vi "Worker Main.vi"() -> ()   [LabVIEW 2013, in "VIChallenge.lvlib"]
uses:
  <vilib>/LabVIEW Hacker/VIChallenge/VIChallenge.lvlib
  <vilib>/LabVIEW Hacker/VIChallenge/Public/Worker State.ctl
  <vilib>/LabVIEW Hacker/LVH-Toolbox/Common/LVH-Common.lvlib
  <vilib>/National Instruments/LabVIEW Interface for Amazon S3/LV Interface for Amazon S3.lvlib
panel:
  out "Iterations":i32
  in  "Stop Button":bool
  out "Error Out":errorcluster
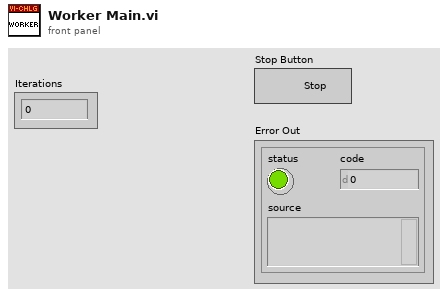
[diagram p1: front panel]
types:
  T1 = typedef "VIChallenge.lvlib/Worker State.ctl" = enum16{"Poll For Job", "Get Source", "Grade", "Notify User"}
  T2 = typedef "VIChallenge.lvlib/VIChallenge Config.ctl" = cluster{"AWS Credentials":T3, "AWS Account Number":string, "SQS Jobs":refnum<class "AWS_SQS.lvclass">, "SQS Status":refnum<class "AWS_SQS.lvclass">, "Source Dir":path, "Working Dir":path, "Output Dir":path, "Archive Dir":path, "job":T4, "Database Ref":T5, "Challenge Dir":path, "Challenges":T6[]}
  T3 = typedef "AWS_Core.lvlib/AWS_AWS Credentials.ctl" = cluster{"AWSAccessKeyId":string, "Secret Key":string}
  T4 = typedef "VIChallenge.lvlib/JSON_job.ctl" = cluster{"job_id":string, "challenge_id":string, "user_id":string, "s3_source_bucket":string, "s3_source_directory":string, "s3_source_filename":string, "status_queue_name":string, "username":string}
  T5 = typedef "NI_Database_API.lvlib/Conn ObjectReference.ctl" = refnum<k1>
  T6 = typedef "VIChallenge.lvlib/Challenge.ctl" = cluster{"General":cluster{"Challenge Id":i32, "Template Path":path, "Solution Path":path, "Primary Score":string, "Score Sort":string}, "Unit Test Framework":cluster{"Enabled Unit Test Templates":path[]}, "VI Analyzer":cluster{"Enabled VI Analyzer Tests":path[]}, "Custom Tests":cluster{"Enabled Custom Tests":path[]}}
  T7 = enum16{"open", "replace", "create", "open or create", "replace or create", "replace or create with confirmation"}
  T8 = typedef "VIChallenge.lvlib/Grader Result.ctl" = cluster{"Id":string, "Score":T9}
  T9 = typedef "VIChallenge.lvlib/Score.ctl" = cluster{"Status":T10, "cpu_time":i32, "max_memory":i32, "style_score":i32, "score0":string, "score1":string, "score2":string, "score3":string, "score4":string, "score5":string}
  T10 = typedef "VIChallenge.lvlib/UTF Status.ctl" = enum16{"Null", "Passed", "Failed", "Error", "Skipped", "Not Processed"}
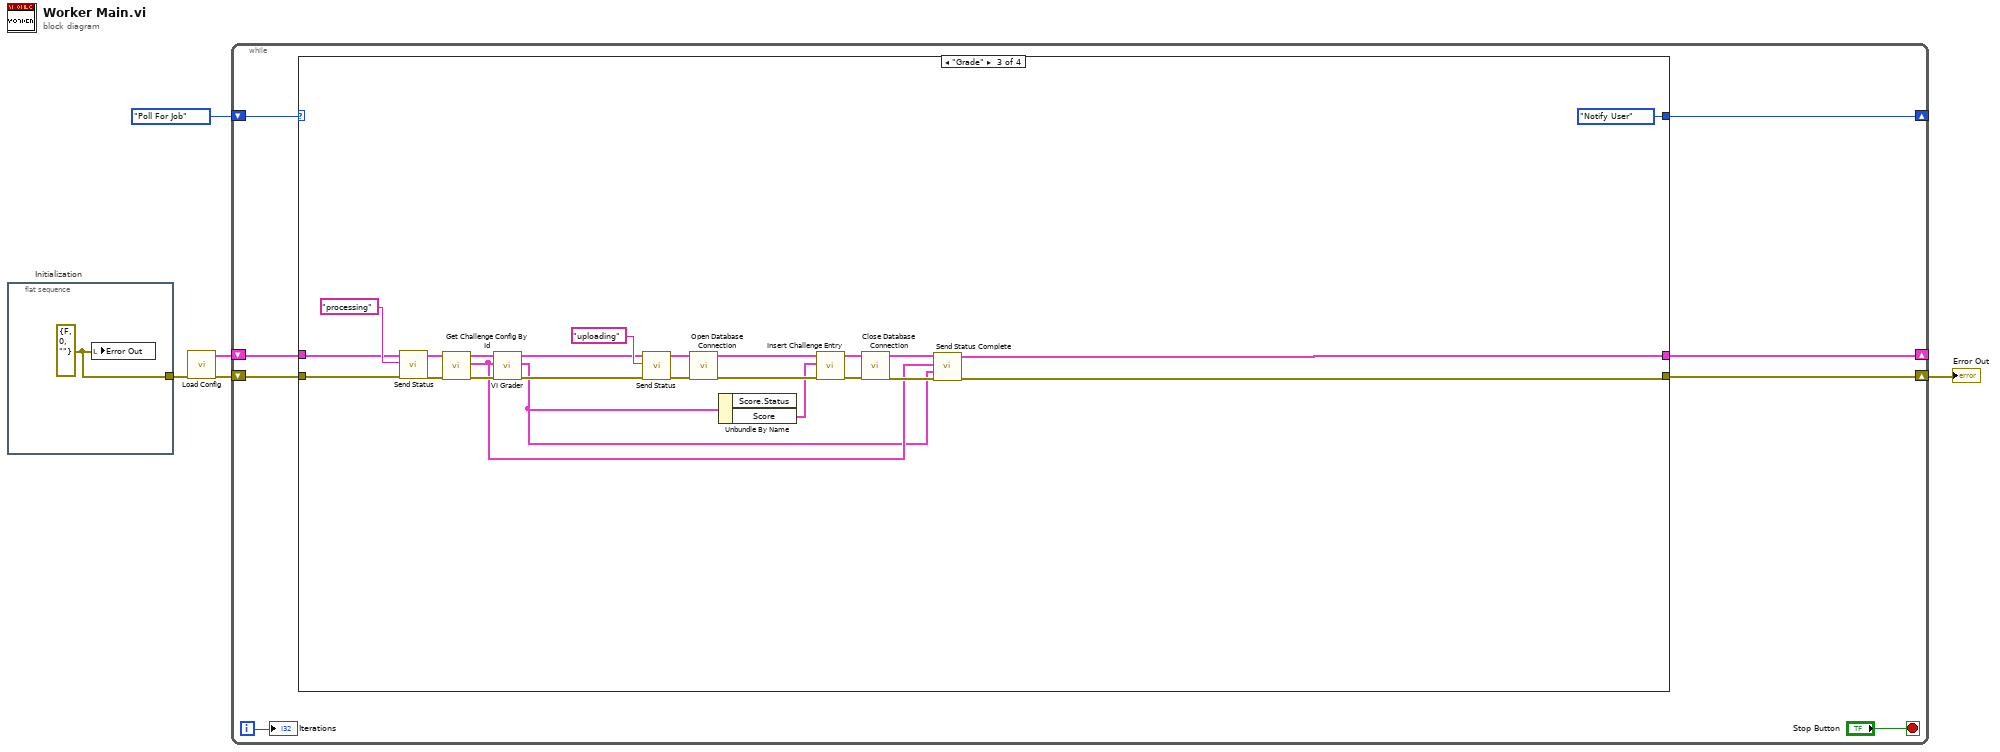
[diagram p0: block diagram]
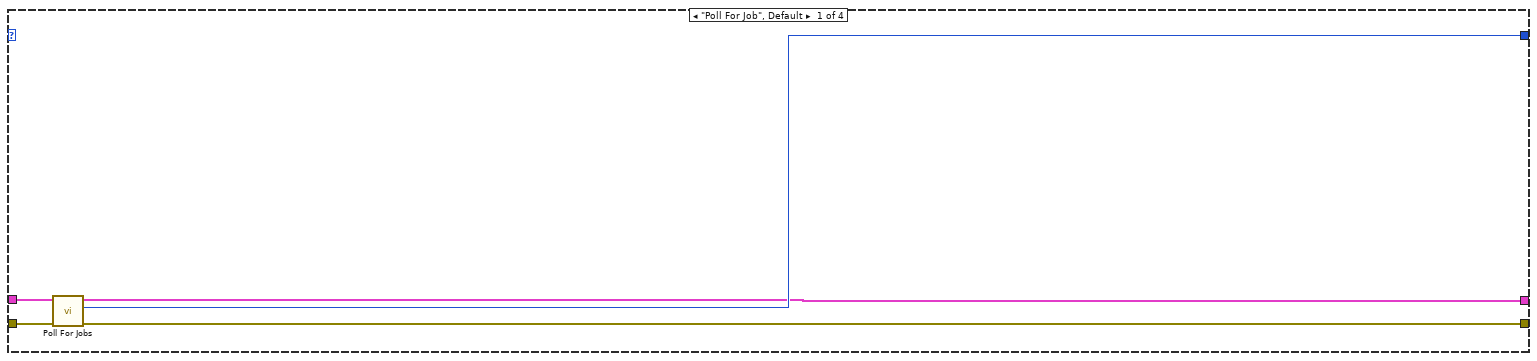
[diagram p2: hidden frame]
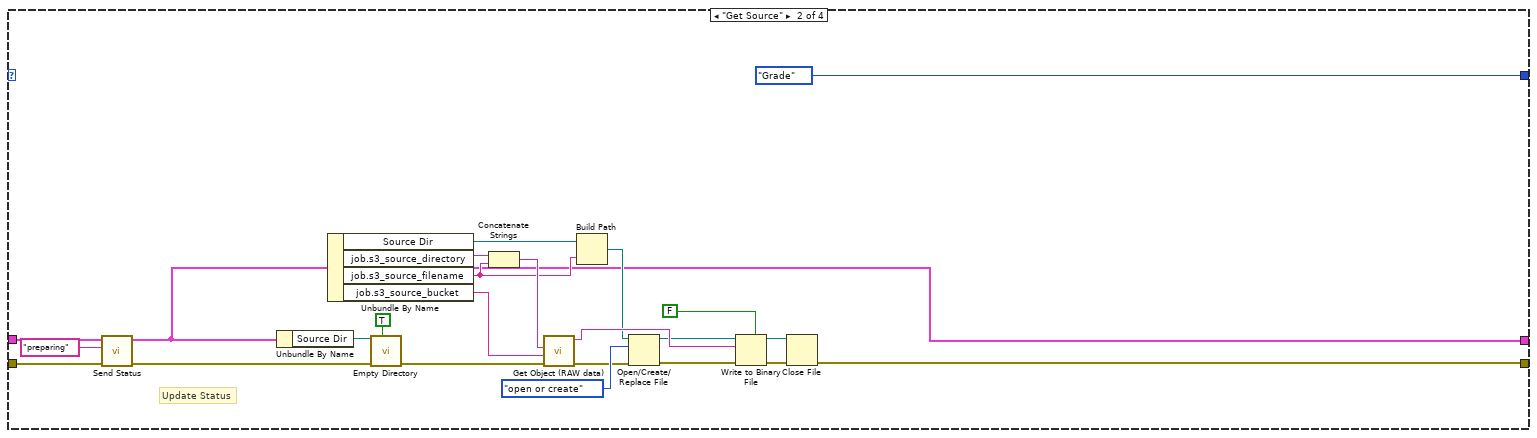
[diagram p3: hidden frame]
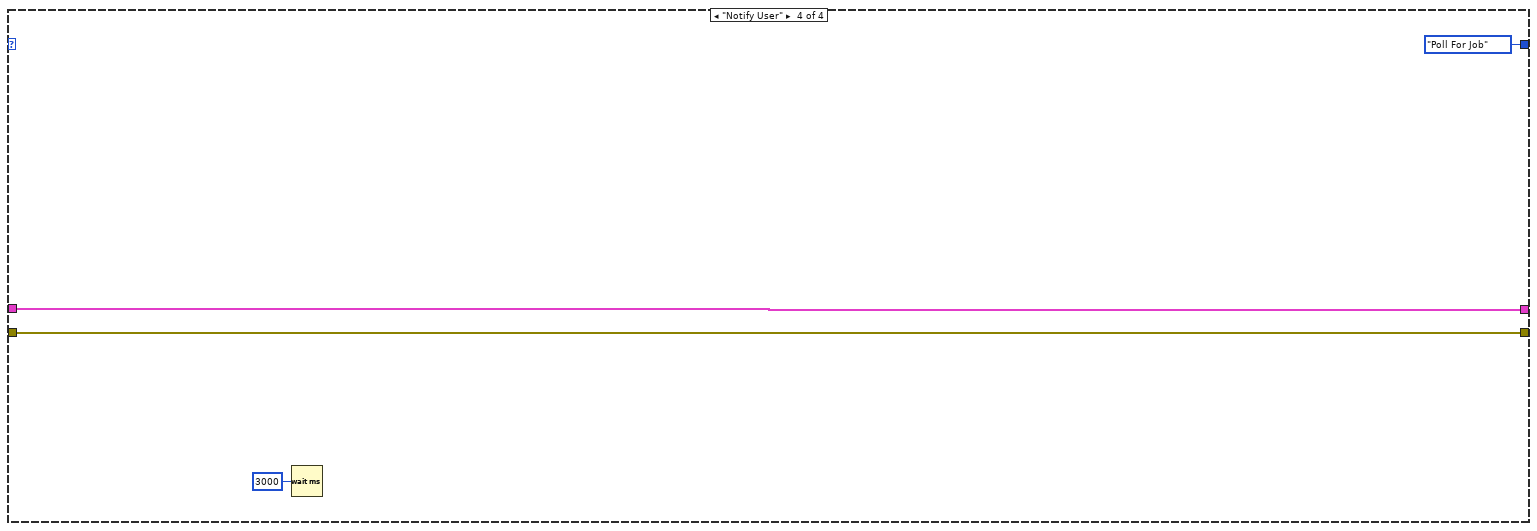
[diagram p4: hidden frame]
diagram:
  n1 = flat-sequence "Initialization" {
    tunnel: [w6] -> w3
    frame #0 {
      w6 = errorcluster {"status"=FALSE, "code"=0, "source"=""} ("Error Out")
      n2 = local write "Error Out"(w6) -> ()
    }
  }
  n3 = call <vilib>:"Load Config.vi"("Error In"=w3) -> ("Error Out"=w2:errorcluster, "VIChallenge Config"=w1:T2)  [unwired: 9 in]
  n4 = while {
    shift-right: [w12] -> w4
    shift-left: w2 -> [w13]
    shift-right: [w7] -> _
    shift-left: Worker_State."Poll For Job" ("Worker State") -> [w14]
    shift-right: [w10] -> _
    shift-left: w1 -> [w11]
    i -> [w8]
    stop <- "Stop Button" stop-if-true
    n5 = case shown="\"Grade\"" w14 {
      tunnel: w13 -> [w19 w23 w66 w68]
      tunnel: [w18 w26 w45 w68] -> w12
      tunnel: w11 -> [w17 w22 w60 w69]
      tunnel: [w15 w21 w44 w69] -> w10
      tunnel: [w16 Worker_State."Grade" ("Worker State") Worker_State."Notify User" ("Worker State") Worker_State."Poll For Job" ("Worker State")] -> w7
      frame "Poll For Job", Default {
        n6 = call <vilib>:"Poll For Jobs.vi"("Error In"=w19, "VIChallenge Config in"=w17) -> ("Error Ou"=w18:errorcluster, "Worker State"=w16:T1, "VIChallenge Config out"=w15:T2)  [unwired: 7 in]
      }
      frame "Get Source" {
        # "Update Status"
        n7 = call <vilib>:"Send Status.vi"("Error In"=w23, "Status"="preparing", "VIChallenge Config"=w22) -> ("Error Out"=w24:errorcluster, "VIChallenge Config"=w21:T2)  [unwired: 7 in]
        n8 = Unbundle By Name(w21) -> ("Source Dir"=w42:path)
        n9 = Unbundle By Name(w21) -> ("Source Dir"=w28:path, "job.s3_source_directory"=w30:string, "job.s3_source_filename"=w27:string, "job.s3_source_bucket"=w31:string)
        n10 = call <vilib>:"Empty Directory.vi"("Delete Files Without Prompt? (F)"=TRUE, "Error In"=w24, "Directory"=w42) -> ("Error Out"=w32:errorcluster)  [unwired: 6 in, 2 out]
        n11 = Concatenate Strings(w30, w27) -> (w29:string)
        n12 = call <vilib>:"Get Object (RAW data).vi"("error in (no error)"=w32, "Bucket"=w31, "Path"=w29) -> ("error out"=w35:errorcluster, "Data"=w39:string)  [unwired: 6 in, 1 out]
        n13 = Build Path(base path=w28, name or relative path=w27) -> (appended path=w36:path)
        n14 = Open/Create/Replace File(file path (use dialog)=w36, error in=w35, operation (0:open)=T7."open or create") -> (refnum out=w37:refnum<file>, error out=w33:errorcluster)  [unwired: 3 in, 1 out]
        n15 = Write to Binary File(file (use dialog)=w37, data=w39, error in=w33, 5:FALSE ("prepend array or string size? (T)")) -> (refnum out=w38:refnum<file>, error out=w34:errorcluster)  [unwired: 2 in, 1 out]
        n16 = Close File(refnum=w38, error in=w34) -> (error out=w26:errorcluster)  [unwired: 1 out]
      }
      frame "Grade" {
        n17 = call <vilib>:"Send Status.vi"("Error In"=w66, "Status"="processing", "VIChallenge Config"=w60) -> ("Error Out"=w63:errorcluster, "VIChallenge Config"=w64:T2)  [unwired: 7 in]
        n18 = call <vilib>:"Get Challenge Config By Id.vi"("Error In"=w63, "VIChallenge Config"=w64) -> ("Error Out"=w62:errorcluster, "Challenge Config"=w47:T6, "VIChallenge Config"=w61:T2)  [unwired: 7 in]
        n19 = call <vilib>:"VI Grader.vi"("Error In"=w62, "Challenge Config"=w47, "VIChallenge Config"=w61) -> ("Error Out"=w53:errorcluster, "Grader Result"=w46:T8, "VIChallenge Config"=w52:T2)  [unwired: 6 in]
        n20 = call <vilib>:"Send Status.vi"("Error In"=w53, "Status"="uploading", "VIChallenge Config"=w52) -> ("Error Out"=w58:errorcluster, "VIChallenge Config"=w57:T2)  [unwired: 7 in]
        n21 = call <vilib>:"Open Database Connection.vi"("Error In"=w58, "VIChallenge Config"=w57) -> ("Error Out"=w56:errorcluster, "VIChallenge Config"=w50:T2)  [unwired: 8 in]
        n22 = Unbundle By Name(w46) -> ("Score"=w51:T9)  [unwired: 1 out]
        n23 = call <vilib>:"Insert Challenge Entry.vi"("Error In"=w56, "Score"=w51, "VIChallenge Config"=w50) -> ("Error Out"=w54:errorcluster, "VIChallenge Config"=w55:T2)  [unwired: 7 in]
        n24 = call <vilib>:"Close Database Connection.vi"("Error In"=w54, "VIChallenge Config"=w55) -> ("Error Out"=w48:errorcluster, "VIChallenge Config"=w49:T2)  [unwired: 8 in]
        n25 = call <vilib>:"Send Status Complete.vi"("Error In"=w48, "Grader Result"=w46, "Challenge Config"=w47, "VIChallenge Config in"=w49) -> ("Error Out"=w45:errorcluster, "VIChallenge Config"=w44:T2)  [unwired: 6 in]
      }
      frame "Notify User" {
        n26 = Wait (ms)(milliseconds to wait=u32 3000) -> ()  [unwired: 1 out]
      }
    }
    "Iterations" <- w8
  }
  "Error Out" <- w4
